vi "VSI Close Device.vi"(10 "DevIndex":i32, 11 "DevType":i32) -> (3 "function return":i32)   [LabVIEW 2010, in "ControlSPI.lvlib"]
doc: "int WINAPI VSI_CloseDevice(int DevType,int DevIndex);"
uses:
  ControlSPI.lvlib
  ControlSPI/Ginkgo_Driver.dll
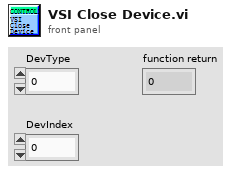
[diagram p1: front panel]
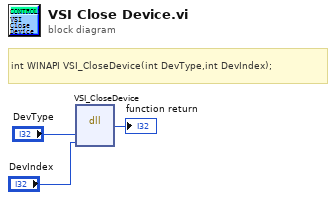
[diagram p0: block diagram]
diagram:
  # "int WINAPI VSI_CloseDevice(int DevType,int DevIndex);"
  n1 = dll-call lib="E:/Project/vt_ginkgo/truck/Ginkgo Driver/vs2010/Ginkgo_USB-I2C&SPI&CAN_API_v2.0.3.3/lib/labview_32bit/ControlSPI/Ginkgo_Driver.*" fn="VSI_CloseDevice"("DevType"="DevType", "DevIndex"="DevIndex") -> (→"function return":i32)  [unwired: 5 in, 2 out]
